vi "Shooter_Teleop.vi"(11 "Joystick_IN":T1={"Pilot Left Joystick X"=0.0, "Pilot Left Joystick Y"=-0.0, "Pilot A Button"=FALSE, "Pilot B Button"=FALSE, "Pilot X Button"=FALSE, "Pilot Y Button"=FALSE, "Pilot Left Bumper"=FALSE, "Pilot Right Bumper"=FALSE, "Pilot View Button"=FALSE, "Pilot Menu Button"=FALSE, "Pilot Left Joystick Press"=FALSE, "Pilot Right Joystick Press"=FALSE, "Pilot Left Trigger"=0.0, "Pilot Right Joystick X"=0.0, "Pilot Right Joystick Y"=0.0, "Pilot Right Trigger"=0.0, "Copilot Left Joystick X"=0.0, "Copilot Left Joystick Y"=0.0, "Copilot A Button"=FALSE, "Copilot B Button"=FALSE, "Copilot X Button"=FALSE, "Copilot Y Button"=FALSE, "Copilot Left Bumper"=FALSE, "Copilot Right Bumper"=FALSE, "Copilot View Button"=FALSE, "Copilot Menu Button"=FALSE, "Copilot Left Joystick Press"=FALSE, "Copilot Right Joystick Press"=FALSE, "Copilot Left Trigger"=0.0, "Copilot Right Joystick X"=0.0, "Copilot Right Joystick Y"=0.0, "Copilot Right Trigger"=0.0, "Pilot D-pad North"=FALSE, "Pilot D-pad South"=FALSE, "Pilot D-pad East"=FALSE, "Pilot D-pad West"=FALSE, "Pilot D-pad NE "=FALSE, "Pilot D-pad SE"=FALSE, "Pilot D-pad SW"=FALSE, "Pilot D-pad NW"=FALSE, "CoPilot D-pad North"=FALSE, "CoPilot D-pad South"=FALSE, "CoPilot D-pad East"=FALSE, "CoPilot D-pad West"=FALSE, "CoPilot D-pad NE"=FALSE, "CoPilot D-pad SE"=FALSE, "CoPilot D-pad SW"=FALSE, "CoPilot D-pad NW"=FALSE, "Pilot Left Trigger Pressed"=FALSE, "Pilot Right Trigger Pressed"=FALSE, "CoPilot Left Trigger Pressed"=FALSE, "CoPilot Right Trigger Pressed"=FALSE}) -> ()   [LabVIEW 2020]
uses:
  Utility VIs/Joystick_Controls.ctl
  Shooter_Cluster.ctl
  Shooter_Control_States.ctl
  Shooter_Globals.vi
  Globals/Turret_Globals.vi
panel:
  in  "toggle reset value":u32=1000
  in  "Deadzone Size":dbl=0.15
  # "e"
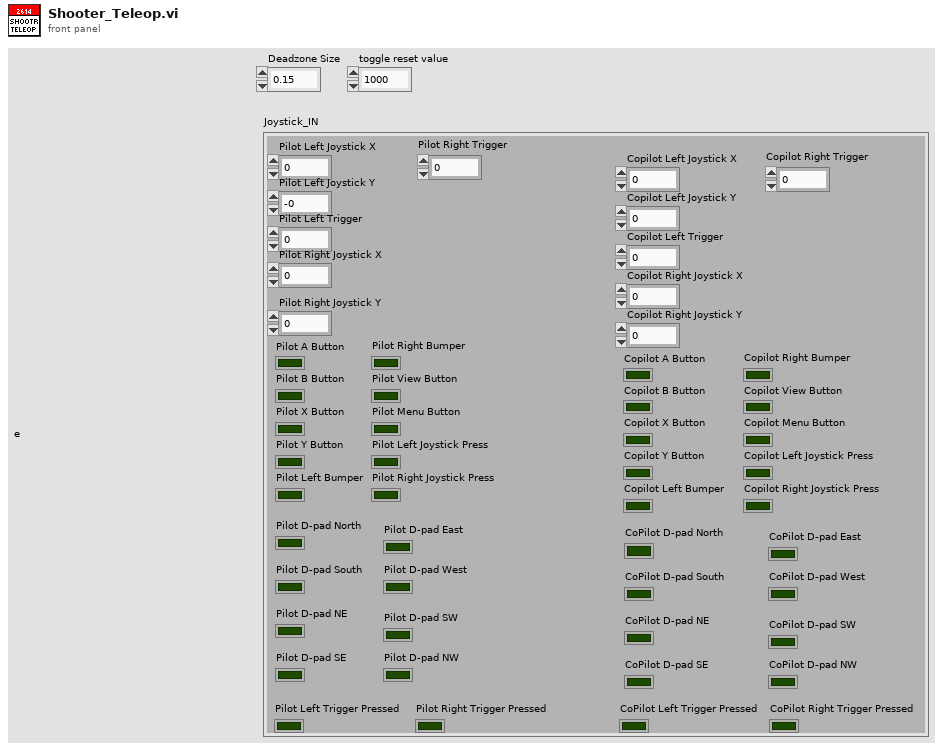
[diagram p1: front panel]
types:
  T1 = typedef "Joystick_Controls.ctl" = cluster{"Pilot Left Joystick X":dbl, "Pilot Left Joystick Y":dbl, "Pilot A Button":bool, "Pilot B Button":bool, "Pilot X Button":bool, "Pilot Y Button":bool, "Pilot Left Bumper":bool, "Pilot Right Bumper":bool, "Pilot View Button":bool, "Pilot Menu Button":bool, "Pilot Left Joystick Press":bool, "Pilot Right Joystick Press":bool, "Pilot Left Trigger":dbl, "Pilot Right Joystick X":dbl, "Pilot Right Joystick Y":dbl, "Pilot Right Trigger":dbl, "Copilot Left Joystick X":dbl, "Copilot Left Joystick Y":dbl, "Copilot A Button":bool, "Copilot B Button":bool, "Copilot X Button":bool, "Copilot Y Button":bool, "Copilot Left Bumper":bool, "Copilot Right Bumper":bool, "Copilot View Button":bool, "Copilot Menu Button":bool, "Copilot Left Joystick Press":bool, "Copilot Right Joystick Press":bool, "Copilot Left Trigger":dbl, "Copilot Right Joystick X":dbl, "Copilot Right Joystick Y":dbl, "Copilot Right Trigger":dbl, "Pilot D-pad North":bool, "Pilot D-pad South":bool, "Pilot D-pad East":bool, "Pilot D-pad West":bool, "Pilot D-pad NE ":bool, "Pilot D-pad SE":bool, "Pilot D-pad SW":bool, "Pilot D-pad NW":bool, "CoPilot D-pad North":bool, "CoPilot D-pad South":bool, "CoPilot D-pad East":bool, "CoPilot D-pad West":bool, "CoPilot D-pad NE":bool, "CoPilot D-pad SE":bool, "CoPilot D-pad SW":bool, "CoPilot D-pad NW":bool, "Pilot Left Trigger Pressed":bool, "Pilot Right Trigger Pressed":bool, "CoPilot Left Trigger Pressed":bool, "CoPilot Right Trigger Pressed":bool}
  T2 = typedef "Shooter_Cluster.ctl" = cluster{"Control_State":T3, "Shooting?":bool, "UpperGoal?":bool, "Limelight?":bool, "Flywheel_%Vbus":dbl, "Cowl_%Vbus":dbl, "Turret_%Vbus":dbl, "Parameters":dbl[], "Auto_Notifier":refnum<notifier>, "Step":i32, "Zero_Turret":bool, "Puke?":bool, "Turret_Target":dbl, "Turret_Manual_Position_Control?":bool, "Turret_Control?":bool, "Turret_Manual_Percent_Control?":bool}
  T3 = typedef "Shooter_Control_States.ctl" = enum16{"No-Op", "Limelight_Shooting", "Shoot_From_Pose", "Test", "Command_Shoot", "Manual", "Puke-Op", "Command_Shoot_From_Pose", "Turret Control", "Turret_Cowl_Zero", "Command_Passive_Flywheel", "Command_Puke_Op"}
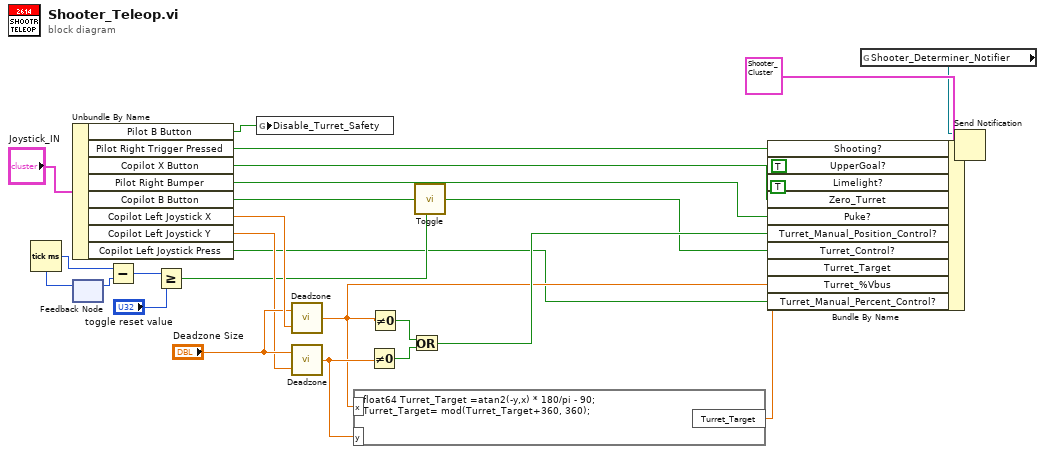
[diagram p0: block diagram]
diagram:
  n1 = Tick Count (ms)() -> (millisecond timer value=w17:u32)
  n2 = Unbundle By Name("Joystick_IN") -> ("Pilot B Button"=w14:bool, "Pilot Right Trigger Pressed"=w26:bool, "Copilot X Button"=w25:bool, "Pilot Right Bumper"=w15:bool, "Copilot B Button"=w5:bool, "Copilot Left Joystick X"=w13:dbl, "Copilot Left Joystick Y"=w11:dbl, "Copilot Left Joystick Press"=w1:bool)
  n3 = feedback #1() -> (w16:u32)  [unwired: 1 in]
  n4 = feedback-in #1(w17) -> ()
  n5 = Subtract(x=w17, y=w16) -> (x-y=w19:u32)
  n6 = Greater Or Equal?(x=w19, y="toggle reset value") -> (x >= y?=w4:bool)
  n7 = global write "Turret_Globals.vi" "Disable_Turret_Safety"(w14) -> ()
  n8 = call "Deadzone.vi"("Joystick Value Input"=w13, "Deadzone Size"="Deadzone Size") -> ("Corrected Joystick Value"=w2:dbl)  [unwired: 1 in]
  n9 = call "Deadzone.vi"("Joystick Value Input"=w11, "Deadzone Size"="Deadzone Size") -> ("Corrected Joystick Value"=w9:dbl)  [unwired: 1 in]
  n10 = formula code="float64 Turret_Target =atan2(-y,x) * 180/pi - 90;\nTurret_Target= mod(Turret_Target+360, 360);"("x"=w2, "y"=w9) -> ("Turret_Target"=w10:dbl)
  n11 = Not Equal To 0?(x=w9) -> (x != 0?=w7:bool)
  n12 = Not Equal To 0?(x=w2) -> (x != 0?=w8:bool)
  n13 = Or(x=w8, y=w7) -> (x .or. y?=w6:bool)
  n14 = call "Toggle.vi"("Boolean"=w5, "reset"=w4) -> ("Boolean Out"=w3:bool)  [unwired: 5 in]
  n15 = Bundle By Name(cluster=T2 {"Control_State"=enum."No-Op", "Shooting?"=FALSE, "UpperGoal?"=FALSE, "Limelight?"=FALSE, "Flywheel_%Vbus"=0.0, "Cowl_%Vbus"=0.0, "Turret_%Vbus"=0.0, "Parameters"=[], "Auto_Notifier"=refnum, "Step"=0, "Zero_Turret"=FALSE, "Puke?"=FALSE, "Turret_Target"=0.0, "Turret_Manual_Position_Control?"=FALSE, "Turret_Control?"=FALSE, "Turret_Manual_Percent_Control?"=FALSE} ("Shooter_Determiner"), "Shooting?"=w26, "UpperGoal?"=TRUE, "Limelight?"=TRUE, "Zero_Turret"=w25, "Puke?"=w15, "Turret_Manual_Position_Control?"=w6, "Turret_Control?"=w3, "Turret_Target"=w10, "Turret_%Vbus"=w2, "Turret_Manual_Percent_Control?"=w1) -> (w27:T2)
  n16 = global read "Shooter_Globals.vi" "Shooter_Determiner_Notifier"() -> (w20:refnum<notifier>)
  n17 = Send Notification(notification=w27, notifier=w20) -> ()  [unwired: 1 in, 2 out]
